vi "Get Current State.vi"(8 "error in (no error)":errorcluster, 11 "VI in":refnum<vi>) -> (0 "error out":errorcluster, 3 "State":variant)   [LabVIEW 2021]
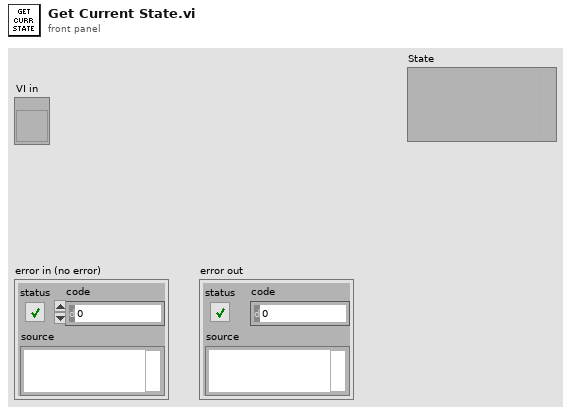
[diagram p1: front panel]
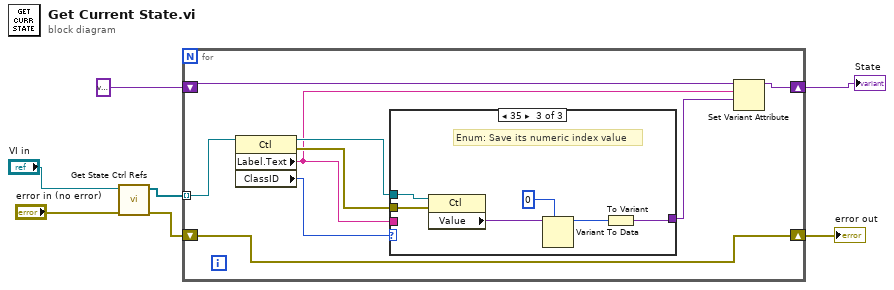
[diagram p0: block diagram]
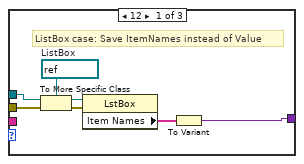
[diagram p2: hidden frame]
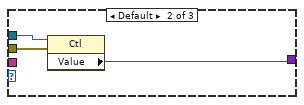
[diagram p3: hidden frame]
diagram:
  n1 = call <vilib>:"Get State Ctrl Refs.vi"("error in (no error)"="error in (no error)", "vi ref"="VI in") -> ("error out"=w6:errorcluster, "All Controls[]"=w5:refnum<vi>[])  [unwired: 8 in]
  n2 = for {
    tunnel: w5 -> [w16] mode=indexing
    shift-right: [w8] -> w7
    shift-left: w6 -> [w8]
    shift-right: [w9] -> w1
    shift-left: variant ("Value") -> [w12]
    n3 = property class="Ctl"(reference=w16) -> (reference out=w15:refnum<vi>, error out=w14:errorcluster, "Label.Text"=w11:string, "ClassID"=w13:u32)  [unwired: 1 in]
    n4 = case shown="35" w13 {
      tunnel: w15 -> [w23 w26 w32]
      tunnel: w14 -> [w18 w25 w31]
      tunnel: w11 -> [_ _ _]
      tunnel: [w17 w24 w27] -> w10
      frame 12 {
        w22 = refnum<vi> refnum  # ListBox
        # "ListBox case: Save ItemNames instead of Value"
        n5 = To More Specific Class(target class=w22, reference=w23, error in=w18) -> (specific class reference=w21:refnum<vi>, error out=w20:errorcluster)
        n6 = property class="LstBox"(reference=w21, error in=w20) -> ("Item Names"=w19:string[])  [unwired: 2 out]
        n7 = To Variant(anything=w19) -> (Variant=w17:variant)
      }
      frame Default {
        n8 = property class="Ctl"(reference=w26, error in=w25) -> ("Value"=w24:variant)  [unwired: 2 out]
      }
      frame 35 {
        # "Enum: Save its numeric index value"
        n9 = property class="Ctl"(reference=w32, error in=w31) -> ("Value"=w30:variant)  [unwired: 2 out]
        n10 = Variant To Data(type=u8 0, Variant=w30) -> (data=w28:u8)  [unwired: 1 in, 1 out]
        n11 = To Variant(anything=w28) -> (Variant=w27:variant)
      }
    }
    n12 = Set Variant Attribute(Variant=w12, name=w11, value=w10) -> (Variant out=w9:variant)  [unwired: 1 in, 2 out]
  }
  "error out" <- w7
  "State" <- w1
